vi "GetDevicesFromMetadata.vi"(8 "error in (no error)":errorcluster, 10 "Title":string, 11 "MetaDataObj in":refnum<class "MetaDataObj.lvclass">) -> (0 "error out":errorcluster, 1 "Found?":bool, 2 "Supported Devices":u32[](array[numeric]), 3 "MetaDataObj Out":refnum<class "MetaDataObj.lvclass">)   [LabVIEW 2021, in "myRIOMetaDataObj.lvclass"]
uses:
  myRIOMetaDataObj.lvclass
  <resource>/dialog/NewProjectWizard/MetaDataObj/MetaDataObj.lvclass
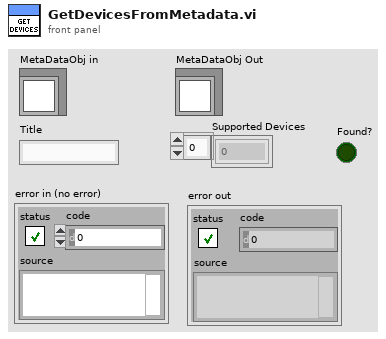
[diagram p1: front panel]
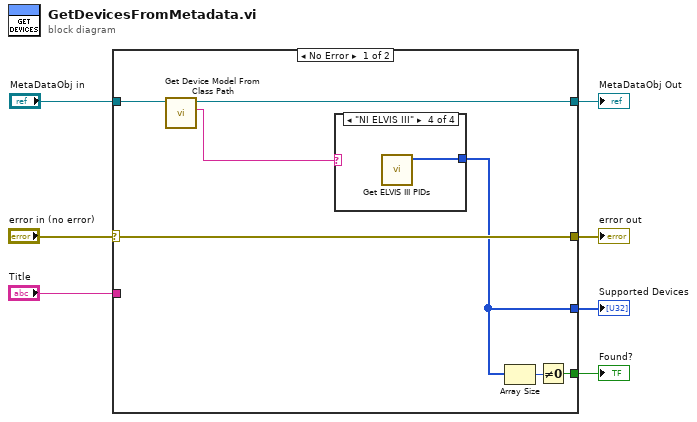
[diagram p0: block diagram]
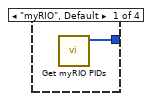
[diagram p2: hidden frame]
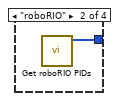
[diagram p3: hidden frame]
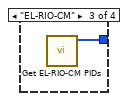
[diagram p4: hidden frame]
diagram:
  n1 = case shown="No Error" "error in (no error)" {
    selector: "error in (no error)" -> [w10 w22]
    tunnel: "Title" -> [_ _]
    tunnel: [w10 w22] -> w6
    tunnel: [w9 FALSE ("selection")] -> w4
    tunnel: [w8 u32[] []] -> w3
    tunnel: "MetaDataObj in" -> [w14 w19]
    tunnel: [w13 w19] -> w1
    frame No Error {
      n2 = call "Get Device Model From Class Path.vi"("MetaDataObj in"=w14) -> ("Device Model Str"=w11:string, "MetaDataObj Out"=w13:refnum<class "MetaDataObj.lvclass">)  [unwired: 8 in, 1 out]
      n3 = case shown="\"NI ELVIS III\"" w11 {
        tunnel: [w15 w16 w17 w18] -> w8
        frame "myRIO", Default {
          n4 = call <vilib>:"Get myRIO PIDs.vi"() -> ("myRIO PIDs"=w15:u32[])  [unwired: 11 in]
        }
        frame "roboRIO" {
          n5 = call <vilib>:"Get roboRIO PIDs.vi"() -> ("roboRIO PIDs"=w16:u32[])  [unwired: 11 in]
        }
        frame "EL-RIO-CM" {
          n6 = call <vilib>:"Get EL-RIO-CM PIDs.vi"() -> ("EL-RIO-CM PIDs"=w17:u32[])  [unwired: 11 in]
        }
        frame "NI ELVIS III" {
          n7 = call <vilib>:"Get ELVIS III PIDs.vi"() -> ("ELVIS III PIDs"=w18:u32[])  [unwired: 11 in]
        }
      }
      n8 = Array Size(array=w8) -> (size(s)=w12:i32)
      n9 = Not Equal To 0?(x=w12) -> (x != 0?=w9:bool)
    }
    frame Error {
      (unwired) FALSE
    }
  }
  "error out" <- w6
  "Found?" <- w4
  "Supported Devices" <- w3
  "MetaDataObj Out" <- w1
